vi "select new configs.vi"(0 "Current Working Dir":path=path "None", 5 "Select New Configs":bool, 9 "App Name":string="data") -> (2 "Open Configs":T1, 3 "New Open Config?":bool, 4 "Working Dir Out":path=path "None", 6 "Exp Configs":T2, 8 "New Exp Config?":bool)   [LabVIEW 2025]
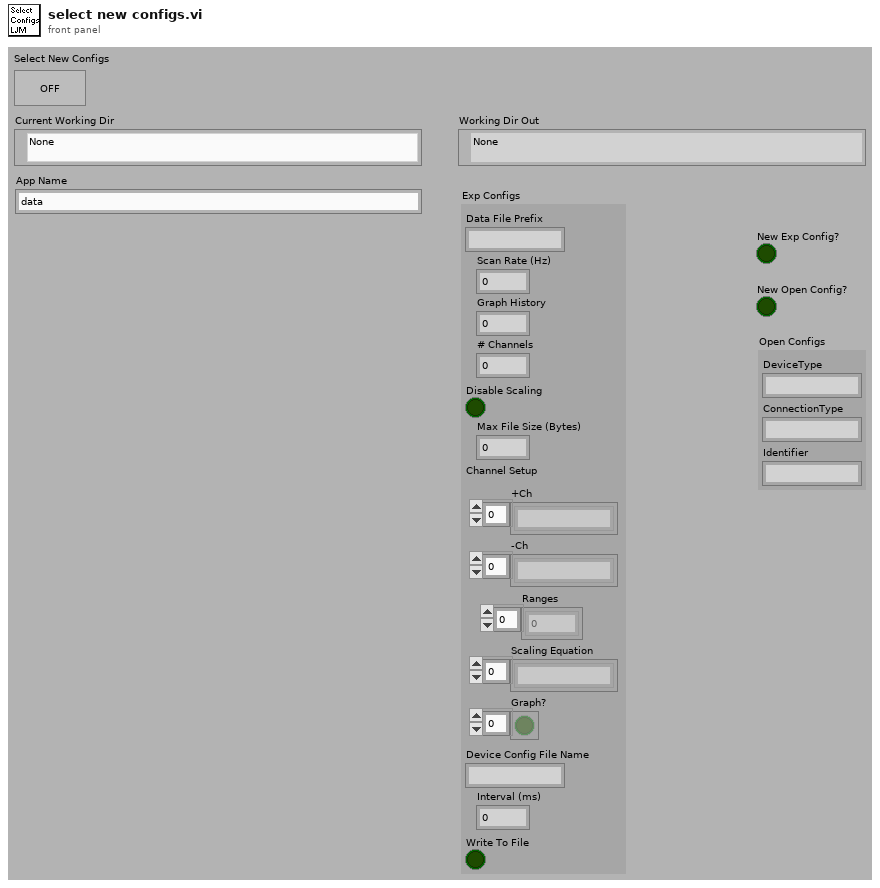
[diagram p1: front panel]
types:
  T1 = cluster{"DeviceType":string, "ConnectionType":string, "Identifier":string}
  T2 = cluster{"Data File Prefix":string, "Scan Rate (Hz)":dbl, "Graph History":i32, "# Channels":i32, "Disable Scaling":bool, "Max File Size (Bytes)":i32, "Channel Setup":cluster{"+Ch":string[], "-Ch":string[], "Ranges":u16[], "Scaling Equation":string[], "Graph?":bool[]}, "Device Config File Name":string, "Interval (ms)":u32, "Write To File":bool}
  T3 = cluster{"+Ch":string[], "-Ch":string[], "Ranges":u16[], "Scaling Equation":string[], "Graph?":bool[]}
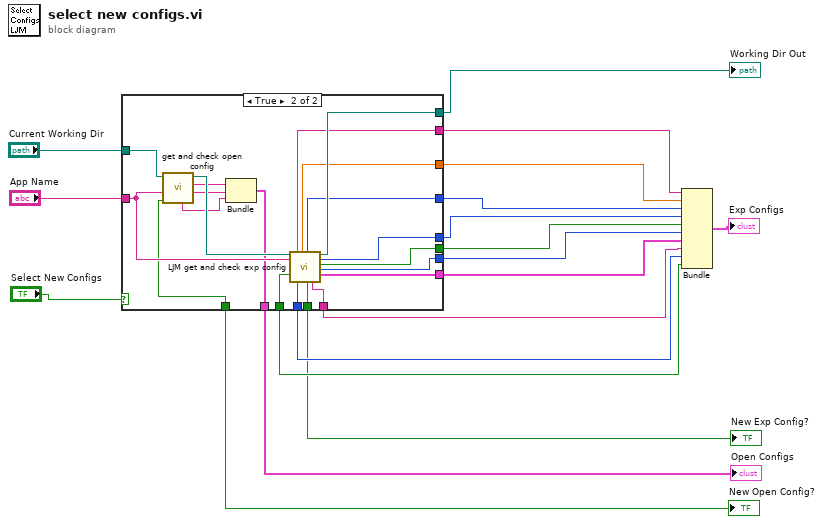
[diagram p0: block diagram]
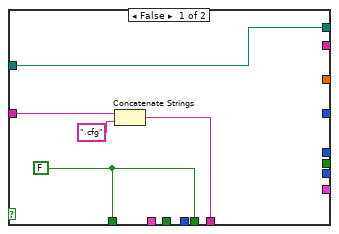
[diagram p2: hidden frame]
diagram:
  n1 = case shown="True" "Select New Configs" {
    tunnel: "Current Working Dir" -> [w23 w29]
    tunnel: "App Name" -> [w21 w42]
    tunnel: [w23 w41] -> w16
    tunnel: [w20 w40] -> w1
    tunnel: [_ w39] -> w15
    tunnel: [_ w38] -> w14
    tunnel: [_ w37] -> w13
    tunnel: [_ w36] -> w12
    tunnel: [_ w34] -> w11
    tunnel: [_ w35] -> w10
    tunnel: [_ w33] -> w9
    tunnel: [_ w32] -> w8
    tunnel: [_ w31] -> w7
    tunnel: [w19 w30] -> w5
    tunnel: [_ w25] -> w4
    tunnel: [w19 w24] -> w3
    frame False {
      w19 = FALSE ("New Exp Config?")
      n2 = Concatenate Strings(w21, ".cfg" ("string")) -> (w20:string)
    }
    frame True {
      n3 = call "get and check open config.vi"("App Name"=w42, "Working Directory In"=w29) -> ("ConnectionType"=w27:string, "DeviceType"=w28:string, "Working Directory Out"=w43:path, "Identifier"=w26:string, "New Open Config?"=w24:bool)  [unwired: 3 in, 2 out]
      n4 = Bundle("DeviceType"=w28, "ConnectionType"=w27, "Identifier"=w26) -> (w25:T1)  [unwired: 1 in]
      n5 = call "LJM get and check exp config.vi"("Working Directory In"=w43, "App Name"=w42) -> ("Write To File"=w31:bool, "Data File Prefix"=w39:string, "Interval (ms)"=w32:u32, "Scan Rate (Hz)"=w38:dbl, "Graph History"=w37:i32, "New Exp Config?"=w30:bool, "Device Config File Name"=w40:string, "Device Config Path"=w41:path, "# Channels"=w36:i32, "Disable Scaling"=w34:bool, "Max File Size (Bytes)"=w35:i32, "Channel Setup"=w33:T3)  [unwired: 5 in, 1 out]
    }
  }
  "Working Dir Out" <- w16
  "New Exp Config?" <- w5
  "Open Configs" <- w4
  "New Open Config?" <- w3
  n6 = Bundle("Data File Prefix"=w15, "Scan Rate (Hz)"=w14, "Graph History"=w13, "# Channels"=w12, "Disable Scaling"=w11, "Max File Size (Bytes)"=w10, "Channel Setup"=w9, "Device Config File Name"=w1, "Interval (ms)"=w8, "Write To File"=w7) -> (→"Exp Configs":T2)  [unwired: 1 in]
